vi "CSDB_Config.get Attribute type.vi"(3 "AttributeName":string, 5 "error in (no error)":errorcluster) -> (17 "Type":string, 19 "error out":errorcluster)   [LabVIEW 2014, in "CSDB_Config.lvlib"]
doc: "Gets the type of an attribute element."
uses:
  CSDB_Config.lvlib
  <vilib>/addons/database/_DB Variant To Data/Database Variant To Data.xnode
  <vilib>/addons/database/NI_Database_API.lvlib
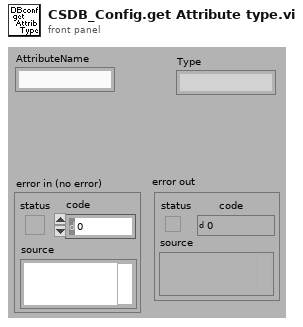
[diagram p1: front panel]
types:
  T1 = typedef "NI_Database_API.lvlib/Conn ObjectReference.ctl" = refnum<k1>
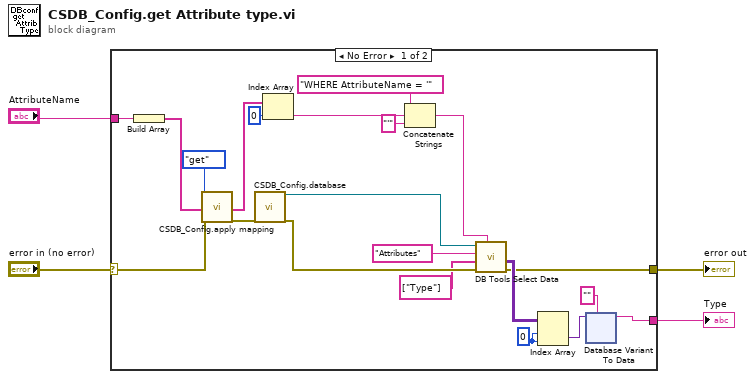
[diagram p0: block diagram]
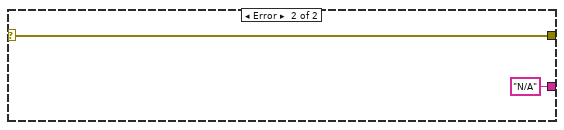
[diagram p2: hidden frame]
diagram:
  n1 = case shown="No Error" "error in (no error)" {
    selector: "error in (no error)" -> [w6 w59]
    tunnel: "AttributeName" -> [w21 _]
    tunnel: [w9 "N/A"] -> w3
    tunnel: [w7 w59] -> w2
    frame No Error {
      w23 = 0 ("index (row)")
      n2 = Build Array(w21) -> (w20:string[])
      n3 = call "CSDB_Config.apply mapping.vi"("Enum"=enum16{"i 2 BP", "BP 2 i", "get"}."get", "AttributeNamesIn"=w20, "error in (no error)"=w6) -> ("AttributeNames out"=w18:string[], "error out"=w22:errorcluster)  [unwired: 14 in, 1 out]
      n4 = call "CSDB_Config.database.vi"("error in (no error)"=w22) -> ("connectionRef out"=w5:T1, "error out"=w15:errorcluster)  [unwired: 17 in]
      n5 = Index Array(array=w18, index=0) -> (element=w19:string)
      n6 = Concatenate Strings("WHERE AttributeName = '", w19, "'" ("string")) -> (w14:string)
      n7 = call <vilib>:"DB Tools Select Data.vi"("condition"=w14, "error in (no error)"=w15, "columns"=string[] ["Type"], "table"="Attributes", "connection reference"=w5) -> ("error out"=w7:errorcluster, "data"=w11:variant[][])  [unwired: 1 in, 1 out]
      n8 = Index Array(array=w11, index (row)=w23, index (col)=w23) -> (element=w10:variant)
      n9 = xnode "Database Variant To Data"("database variant"=w10, "type"="") -> ("data"=w9:string)  [unwired: 1 in, 1 out]
    }
    frame Error {
    }
  }
  "error out" <- w2
  "Type" <- w3
